vi "Send CCD Status.vi"(8 "error in (no error)":errorcluster, 11 "RxTx in":refnum<class "RxTx.lvclass">) -> (0 "error out":errorcluster, 3 "RxTx out":refnum<class "RxTx.lvclass">)   [LabVIEW 2018, in "RxTx.lvclass"]
uses:
  RxTx.lvclass
  RxTx.lvclass/RxTx.ctl
  Interface/Interface.lvclass
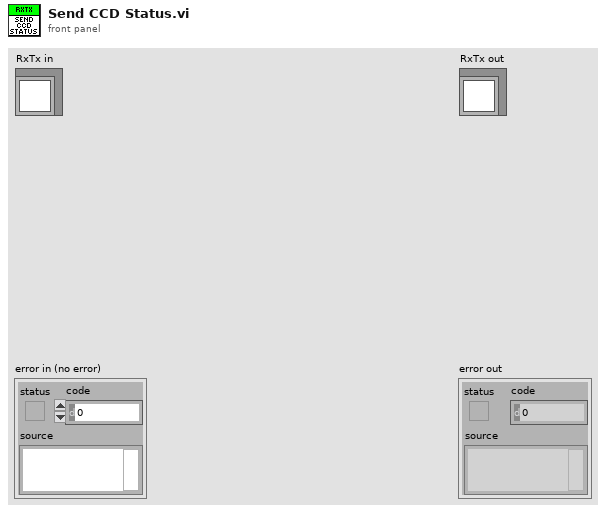
[diagram p1: front panel]
types:
  T1 = cluster{"CUBE_EXPOSURE_TIME":sgl, "CUBES_DONE":u16, "LAST_IMAGE_NAME":string, "DISK_SPACE":u16, "FRAMES_DONE":u16, "CCD_STATUS":string, "CURRENT_TEMPERATURE":i16, "TEMPERATURE_STATUS":string, "FRAME_EXPOSURE_TIME":dbl, "CCD_POWER_STATUS":bool, "SERIAL_NUMBER":u16, "ACQUIRING":bool}
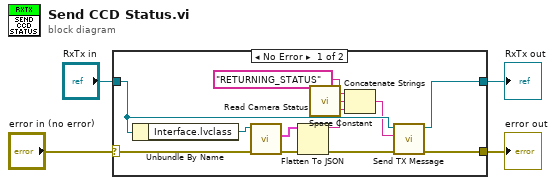
[diagram p0: block diagram]
diagram:
  n1 = case shown="No Error" "error in (no error)" {
    selector: "error in (no error)" -> [w13 w18]
    tunnel: [w5 w18] -> w2
    tunnel: [w7 w17] -> w1
    tunnel: "RxTx in" -> [w12 w17]
    frame No Error {
      n2 = Unbundle By Name(w12) -> ("Interface.lvclass"=w16:refnum<class "Interface.lvclass">)
      n3 = call "Read Camera Status.vi"("error in (no error)"=w13, "Interface in"=w16) -> ("error out"=w10:errorcluster, "Camera Status"=w11:T1)  [unwired: 7 in, 1 out]
      n4 = Flatten To JSON(anything=w11, error in (no error)=w10) -> (JSON string=w8:string, 11:w9:errorcluster)  [unwired: 1 in]
      n5 = call <vilib>:"Space Constant.vi"() -> ("String"=w15:string)
      n6 = Concatenate Strings("RETURNING_STATUS", w15, w8) -> (w6:string)
      n7 = call "Send TX Message.vi"("error in (no error)"=w9, "element"=w6, "RxTx in"=w12) -> ("error out"=w5:errorcluster, "RxTx out"=w7:refnum<class "RxTx.lvclass">)  [unwired: 7 in]
    }
    frame Error {
    }
  }
  "error out" <- w2
  "RxTx out" <- w1
